vi "Invert In-Place (Greyscale Negate).vi"(8 "error in (no error)":errorcluster, 11 "Greyscale Image to Invert in Place in":T1) -> (0 "error out":errorcluster, 3 "Greyscale Image":T1)   [LabVIEW 2020, in "image.lvlib"]
doc: "Invert the Pixels in the Greyscale Image in-place.\n\nThis function is useful when inverting a Greyscale Image which represents a mask."
uses:
  image.lvlib
  Greyscale Image.ctl
  04247039-c0b2-4e2c-ba05-6341c33a4f92.vi
  <vilib>/Utility/error.llb/Error Cluster From Error Code.vi
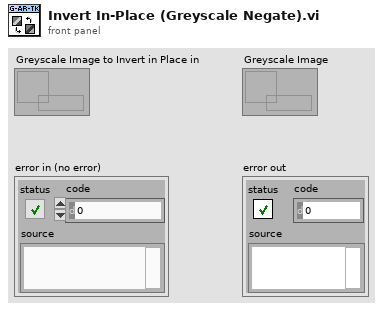
[diagram p1: front panel]
types:
  T1 = typedef "image.lvlib/Greyscale Image.ctl" = refnum<data-value>
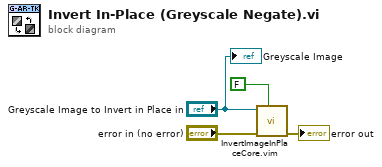
[diagram p0: block diagram]
diagram:
  n1 = call "InvertImageInPlaceCore.vim"("Use Bitwise"=FALSE, "error in (no error)"="error in (no error)", "Image In"="Greyscale Image to Invert in Place in") -> ("error out"=→"error out":errorcluster)  [unwired: 8 in]
  "Greyscale Image" <- "Greyscale Image to Invert in Place in"
